vi "checkDigitalLevel.vi"(10 "Expected":T1, 11 "Actual":bool) -> (3 "Pass?":bool)   [LabVIEW 2015]
uses:
  Typedefs/Digital Signal Level.ctl
  Typedefs/ILCBTTypedefs.lvlib
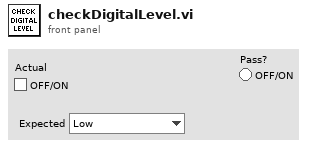
[diagram p1: front panel]
types:
  T1 = typedef "ILCBTTypedefs.lvlib/Digital Signal Level.ctl" = enum16{"Low", "High"}
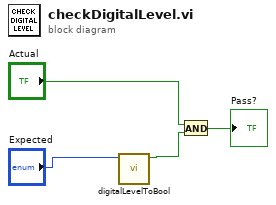
[diagram p0: block diagram]
diagram:
  n1 = call "digitalLevelToBool.vi"("Digital Signal Level"="Expected") -> ("Bool?"=w1:bool)  [unwired: 10 in]
  n2 = And(x="Actual", y=w1) -> (x .and. y?=→"Pass?":bool)
